vi "locate tag to modify.vi"(7 "owner ID":string, 8 "error in":errorcluster, 10 "tag descriptor":refnum<class "tag descriptor.lvclass">, 11 "engine configuration in":refnum<class "engine configuration.lvclass">) -> (0 "error out":errorcluster, 2 "index":i32, 3 "engine configuration out":refnum<class "engine configuration.lvclass">)   [LabVIEW 2013, in "engine configuration.lvclass"]
uses:
  engine configuration.lvclass
  <vilib>/NI/Tag Bus/tag/tag descriptor.lvclass
  engine configuration.lvclass/engine configuration.ctl
  <vilib>/NI/Tag Bus/tag/tag descriptor.lvclass/tag descriptor.ctl
  <vilib>/NI/Tag Bus/tag/read tag name.vi
  <vilib>/NI/Tag Bus Module Framework/root configuration/TBM configuration.lvclass
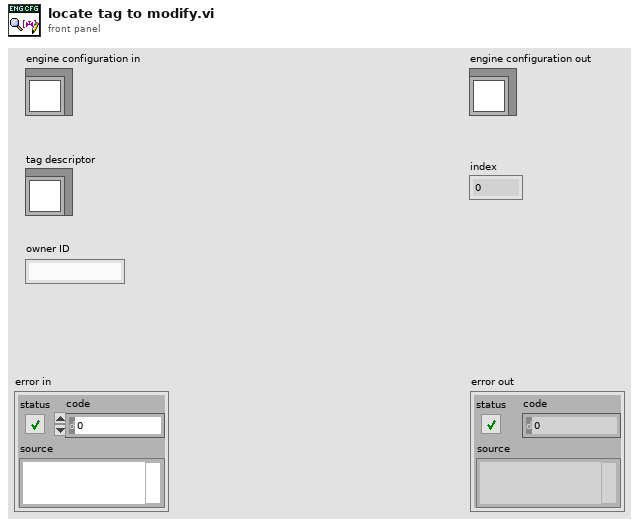
[diagram p1: front panel]
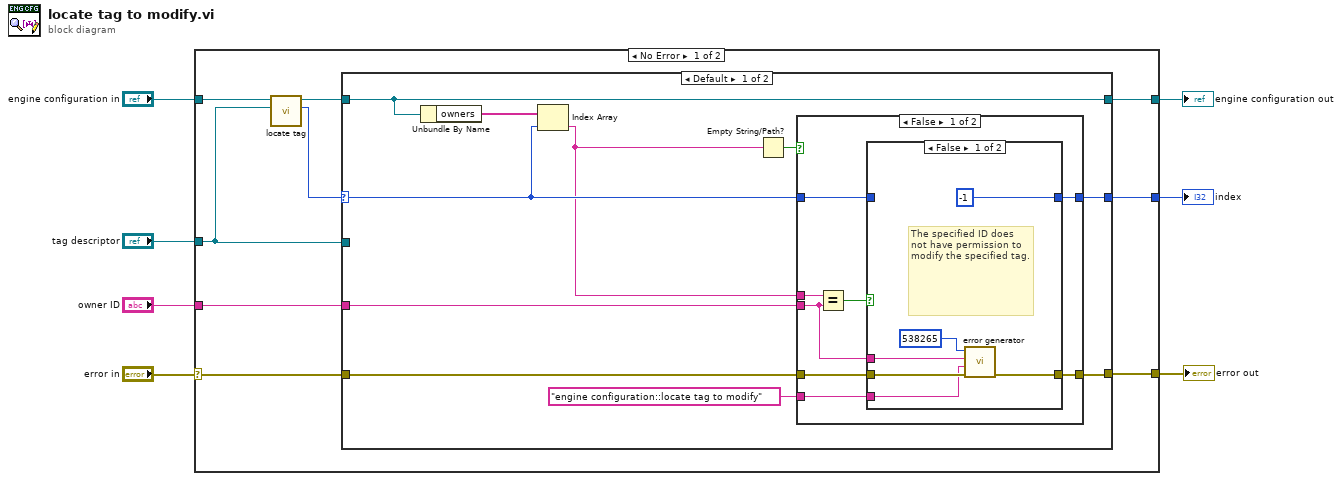
[diagram p0: block diagram]
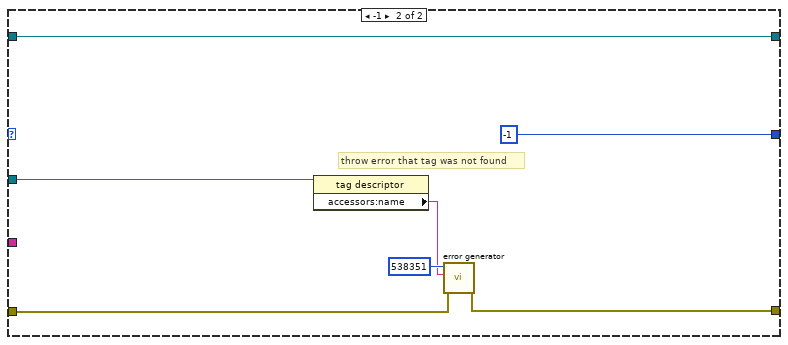
[diagram p4: hidden frame]
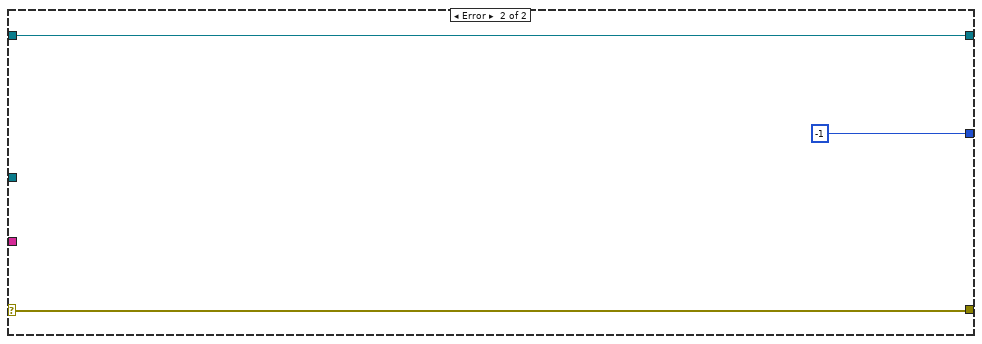
[diagram p5: hidden frame]
diagram:
  n1 = case shown="No Error" "error in" {
    selector: "error in" -> [w12 w52]
    tunnel: "engine configuration in" -> [w16 w54]
    tunnel: [w13 w54] -> w6
    tunnel: "tag descriptor" -> [w11 _]
    tunnel: [w10 w52] -> w3
    tunnel: "owner ID" -> [w9 _]
    tunnel: [w8 -1 ("index")] -> w1
    frame No Error {
      n2 = call "locate tag.vi"("tag descriptor"=w11, "engine configuration in"=w16) -> ("index"=w15:i32, "engine configuration out"=w14:refnum<class "engine configuration.lvclass">)  [unwired: 8 in]
      n3 = case shown="Default" w15 {
        selector: w15 -> [w20 _]
        tunnel: w14 -> [w22 w51]
        tunnel: [w22 w51] -> w13
        tunnel: w12 -> [w24 w49]
        tunnel: w11 -> [_ w48]
        tunnel: [w23 w46] -> w10
        tunnel: w9 -> [w26 _]
        tunnel: [w25 -1 ("index")] -> w8
        frame Default {
          n4 = Unbundle By Name(w22) -> ("owners"=w21:string[])
          n5 = Index Array(array=w21, index=w20) -> (element=w18:string)
          n6 = Empty String/Path?(string/path=w18) -> (empty?=w19:bool)
          n7 = case shown="False" w19 {
            tunnel: w18 -> [w34 _]
            tunnel: w26 -> [w27 _]
            tunnel: w20 -> [w33 w44]
            tunnel: [w32 w44] -> w25
            tunnel: w24 -> [w31 w43]
            tunnel: [w29 w43] -> w23
            tunnel: "engine configuration::locate tag to modify" -> [w28 _]
            frame False {
              n8 = Equal?(x=w34, y=w27) -> (x = y?=w30:bool)
              n9 = case shown="False" w30 {
                tunnel: w33 -> [_ w42]
                tunnel: [-1 ("index") w42] -> w32
                tunnel: w31 -> [w38 w41]
                tunnel: [w37 w41] -> w29
                tunnel: w28 -> [w36 _]
                tunnel: w27 -> [w35 _]
                frame False {
                  # "The specified ID does not have permission to modify the specified tag."
                  n10 = call <vilib>:"error generator.vi"("error in"=w38, "source"=w36, "append error message"=w35, "error code (0)"=538265) -> ("error out"=w37:errorcluster)  [unwired: 7 in]
                }
                frame True {
                }
              }
            }
            frame True {
            }
          }
        }
        frame -1 {
          # "throw error that tag was not found"
          n11 = property class="tag descriptor"(reference=w48) -> ("accessors:name"=w47:string)  [unwired: 1 in, 2 out]
          n12 = call <vilib>:"error generator.vi"("error in"=w49, "append error message"=w47, "error code (0)"=538351) -> ("error out"=w46:errorcluster)  [unwired: 8 in]
        }
      }
    }
    frame Error {
    }
  }
  "engine configuration out" <- w6
  "index" <- w1
  "error out" <- w3
